vi "Position.vi"() -> ()   [LabVIEW 2017]
panel:
  out "Position":i16
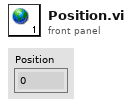
[diagram p1: front panel]
diagram:
